vi "CAN Signal to Frame.vi"(8 "error in (no error)":errorcluster, 9 "Data Array":dbl[](array[numeric]), 10 "Frame":string, 11 "ENET in":refnum<class "ENET_BS1201.lvclass">) -> (0 "error out":errorcluster, 2 "Data":refnum<class "Data.lvclass">, 3 "ENET out":refnum<class "ENET_BS1201.lvclass">)   [LabVIEW 2021]
uses:
  <vilib>/xnet/xnet.llb/XNET Create Session (Conversion).vi
  <vilib>/xnet/xnet.llb/XNET Convert (Signal to Frame CAN).vi
  _Private/Data Classes/CAN Data Class/CAN Data.lvclass
  C:/Users/Public/Documents/Projects/7100-00109 SW BS1201 LV Driver/trunk/source/_Private/Data Classes/Data Class/Data.lvclass
  C:/Users/Public/Documents/Projects/7100-00109 SW BS1201 LV Driver/trunk/source/_Private/Data Classes/CAN Data Class/CAN Data.lvclass
  ENET_BS1201.lvclass
  ENET_BS120x/ENET_BS120x.lvclass
  C:/Users/Public/Documents/Projects/7100-00109 SW BS1201 LV Driver/trunk/source/ENET_BS120x/ENET_BS120x.lvclass
  C:/Users/Public/Documents/Projects/7100-00109 SW BS1201 LV Driver/trunk/source/BS120x.lvclass
  C:/Users/Public/Documents/Projects/7100-00109 SW BS1201 LV Driver/trunk/source/ENET_BS1201/ENET_BS1201.lvclass
  _Private/Data Classes/Data Class/Data.lvclass
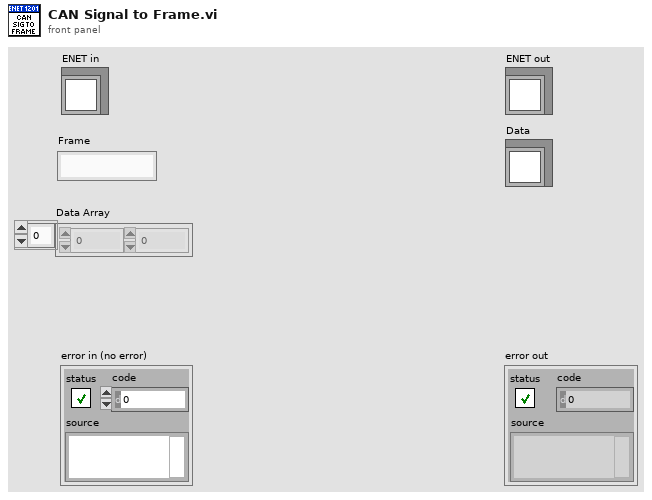
[diagram p1: front panel]
types:
  T1 = cluster{"identifier":u32, "extended?":bool, "type":enum8{"CAN Data", "CAN Remote"}, "payload":u8[]}
  T2 = typedef "XNET Frame CAN.ctl" = cluster{"timestamp":timestamp, "payload":u8[], "identifier":u32, "type":T3, "extended?":bool, "echo?":bool}
  T3 = typedef "XNET Frame Type CAN.ctl" = u8
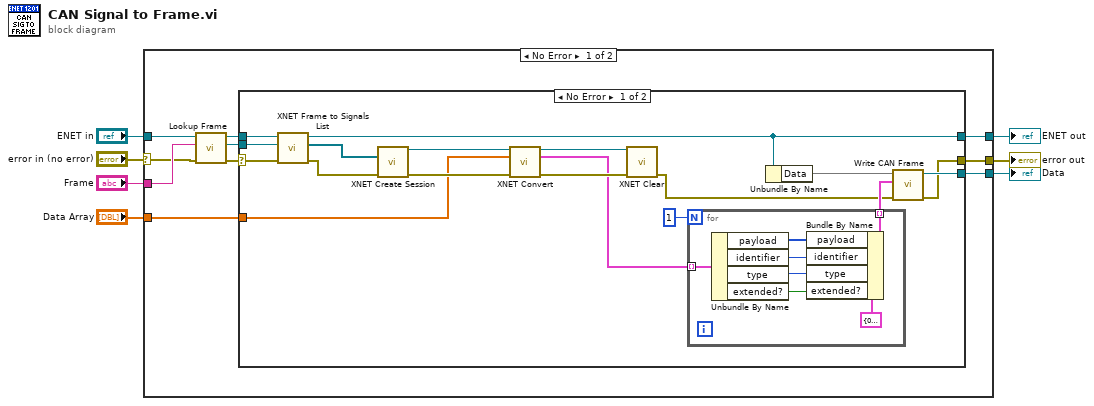
[diagram p0: block diagram]
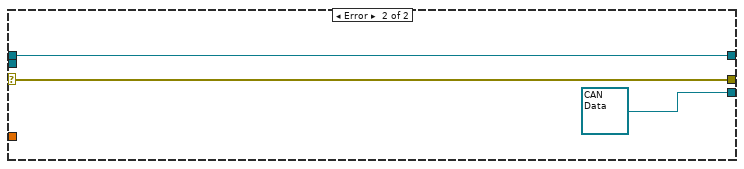
[diagram p2: hidden frame]
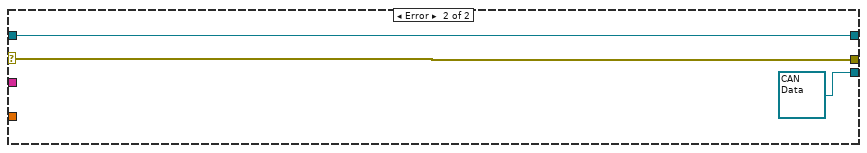
[diagram p3: hidden frame]
diagram:
  n1 = case shown="No Error" "error in (no error)" {
    selector: "error in (no error)" -> [w9 w48]
    tunnel: [w16 w48] -> w4
    tunnel: [w15 w47] -> w1
    tunnel: "ENET in" -> [w13 w47]
    tunnel: "Frame" -> [w10 _]
    tunnel: "Data Array" -> [w17 _]
    tunnel: [w14 refnum<class "CAN Data.lvclass"> refnum ("CAN Data out")] -> w3
    frame No Error {
      n2 = call "Lookup Frame.vi"("error in (no error)"=w9, "Frame"=w10, "Ethernet in"=w13) -> ("error out"=w8:errorcluster, "XNET Frame"=w11:refnum<k21>, "Ethernet out"=w12:refnum<class "ENET_BS1201.lvclass">)  [unwired: 6 in]
      n3 = case shown="No Error" w8 {
        selector: w8 -> [w25 w43]
        tunnel: [w26 w43] -> w16
        tunnel: w17 -> [w33 _]
        tunnel: w12 -> [w21 w45]
        tunnel: [w19 w45] -> w15
        tunnel: [w27 refnum<class "CAN Data.lvclass"> refnum ("CAN Data out")] -> w14
        tunnel: w11 -> [w20 _]
        frame No Error {
          # "CAN frame found"
          n4 = call-dynamic "XNET Frame to Signals List.vi"("error in (no error)"=w25, "XNET Frame"=w20, "BS1200 in"=w21) -> ("error out"=w24:errorcluster, "Sorted XNET Signals"=w22:refnum<k21>[], "BS1200 out"=w19:refnum<class "ENET_BS1201.lvclass">)  [unwired: 6 in]
          n5 = call-poly <vilib>:"XNET Create Session.vi"("signal list"=w22, "error in (no error)"=w24) -> ("session out"=w35:refnum<k21>, "error out"=w34:errorcluster)  [unwired: 12 out]
          n6 = call-poly <vilib>:"XNET Convert.vi"("session in"=w35, "signal data"=w33, "error in (no error)"=w34) -> ("session out"=w32:refnum<k21>, "frame data"=w30:T2[], "error out"=w31:errorcluster)  [unwired: 10 out]
          n7 = call <vilib>:"XNET Clear.vi"("session in"=w32, "error in (no error)"=w31) -> ("error out"=w23:errorcluster)  [unwired: 13 in]
          n8 = for {
            N: 1 -> [_]
            tunnel: w30 -> [w38] mode=indexing
            tunnel: [w37] -> w29 mode=indexing
            n9 = Unbundle By Name(w38) -> ("payload"=w39:u8[], "identifier"=w40:u32, "type"=w41:T3, "extended?"=w42:bool)
            n10 = Bundle By Name(cluster=T1 {"identifier"=0, "extended?"=FALSE, "type"=enum."CAN Data", "payload"=[0, 0, 0, 0, 0, 0, 0, 0]} ("CAN Frame"), "payload"=w39, "identifier"=w40, "type"=w41, "extended?"=w42) -> (w37:T1)
          }
          n11 = Unbundle By Name(w19) -> ("Data"=w18)
          n12 = call "Write CAN Frame.vi"("error in (no error)"=w23, "CAN Frame Array"=w29, "CAN Data in"=w18) -> ("error out"=w26:errorcluster, "CAN Data out"=w27:refnum<class "CAN Data.lvclass">)  [unwired: 7 in]
        }
        frame Error {
          # "CAN Frame not found"
        }
      }
    }
    frame Error {
    }
  }
  "error out" <- w4
  "Data" <- w3
  "ENET out" <- w1
